vi "Write Value (variant).vi"(8 "error in (no error)":errorcluster, 10 "Variant":variant, 11 "U8 D Element in":refnum<class "U8 D Element.lvclass">) -> (0 "error out":errorcluster, 3 "U8 D Element out":refnum<class "U8 D Element.lvclass">)   [LabVIEW 2018, in "D Datagrid Library.lvlib" / "U8 D Element.lvclass"]
uses:
  U8 D Element.lvclass
  U8 D Element.lvclass/U8 D Element.ctl
  Write Value.vi
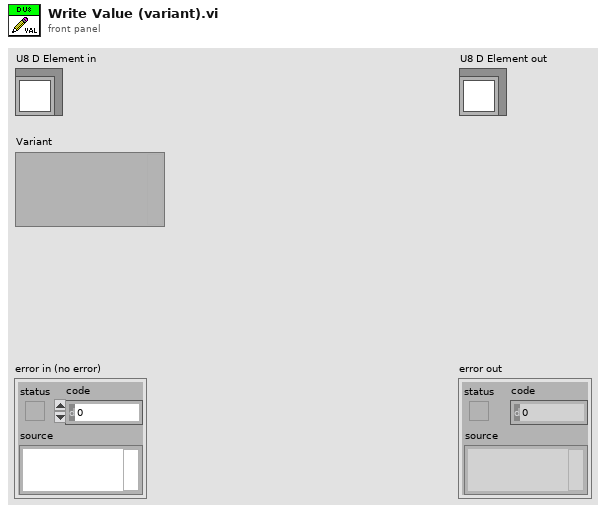
[diagram p1: front panel]
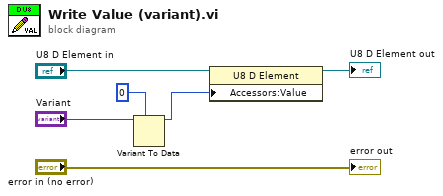
[diagram p0: block diagram]
diagram:
  n1 = Variant To Data(type=u8 0 ("Value"), Variant="Variant") -> (data=w1:u8)  [unwired: 1 in, 1 out]
  n2 = property class="U8 D Element"(reference="U8 D Element in", "Accessors:Value"=w1) -> (reference out=→"U8 D Element out":refnum<class "U8 D Element.lvclass">)  [unwired: 1 in, 1 out]
  "error out" <- "error in (no error)"
